vi "Main.vi"(11 "Module Admin":refnum<class "Delacor_lib_QMH_Module Admin.lvclass">) -> ()   [LabVIEW 2020, in "User Interface.lvlib"]
doc: "This template is based off of the Queued Message Handler design pattern and the Queued Message Handler project template that ships with LabVIEW.\n\nThe main difference is that the queue is private to this module and communication between modules is performed via Broadcast and Request events.\n\nRequest events are wrapped in public API methods and are handled in the Event Handling Loop (EHL) of this VI. Any module can register for Broadcast events sent by this module. The EHL generates messages based on user interface actions.\n\nThe Message Handling Loop (MHL) processes messages generated by the EHL, or by other messages. The messages are string values, so new messages can be added easily to the Message Cases case structure in the MHL. Each message cluster can also provide an optional value for Message Data, which is a variant that can be converted to whatever message-specific data is required.\n_____\nBased on DQMH Project Template 6.1.0.94."
uses:
  User Interface.lvlib
  <vilib>/Delacor/Delacor QMH/Libraries/Module Admin_class/Delacor_lib_QMH_Module Admin.lvclass
  Module Data--cluster.ctl
  Stop Argument--cluster.ctl
  <vilib>/Delacor/Delacor QMH/Libraries/Message Queue_class/Delacor_lib_QMH_Message Queue.lvclass/Delacor_lib_QMH_Message Queue.ctl
  <vilib>/Delacor/Delacor QMH/Libraries/Module Admin_class/Delacor_lib_QMH_Module Admin.lvclass/Delacor_lib_QMH_Module Admin.ctl
  <vilib>/Delacor/Delacor QMH/Libraries/Message Queue_class/Delacor_lib_QMH_Enqueue Message (Single).vi
  <vilib>/Delacor/Delacor QMH/Libraries/Module Admin_class/Delacor_lib_QMH_Get External Launch.vi
  <vilib>/Utility/error.llb/Error Cluster From Error Code.vi
  <vilib>/ErrorRing/Error Ring.xnode
  <vilib>/Delacor/Delacor QMH/Libraries/Message Queue_class/Delacor_lib_QMH_Message Queue.lvclass
  Interface Change/Interface Change.lvlib
panel:
  in  "Close Panel Interface CH":bool
  in  "Open Panel Interface CH":bool
  in  "Color Box":u32(colorbox)
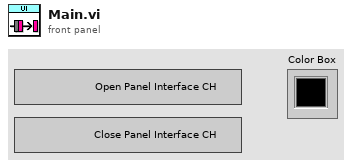
[diagram p1: front panel]
types:
  T1 = typedef "User Interface.lvlib/Request Events--cluster.ctl" = cluster{"Stop Module":refnum<user-event>, "Show Panel":refnum<user-event>, "Hide Panel":refnum<user-event>, "Get Module Execution Status":refnum<user-event>, "Show Diagram":refnum<user-event>}
  T2 = typedef "Interface Change.lvlib/Broadcast Events--cluster.ctl" = cluster{"Module Did Init":refnum<user-event>, "Status Updated":refnum<user-event>, "Error Reported":refnum<user-event>, "Module Did Stop":refnum<user-event>, "Update Module Execution Status":refnum<user-event>}
  T3 = typedef "User Interface.lvlib/Module Data--cluster.ctl" = cluster{"Status":string}
  T4 = enum32{"invalid lock state", "Not Locked", "Locked (No Password)", "Password-protected"}
  T5 = typedef "User Interface.lvlib/Stop Argument--cluster.ctl" = cluster{"Origin":string, "Exit via Stop Module Req?":bool, "Wait for Module to stop?":bool}
  T6 = enum32{"Invalid", "Standard", "Closed", "Hidden", "Minimized", "Maximized"}
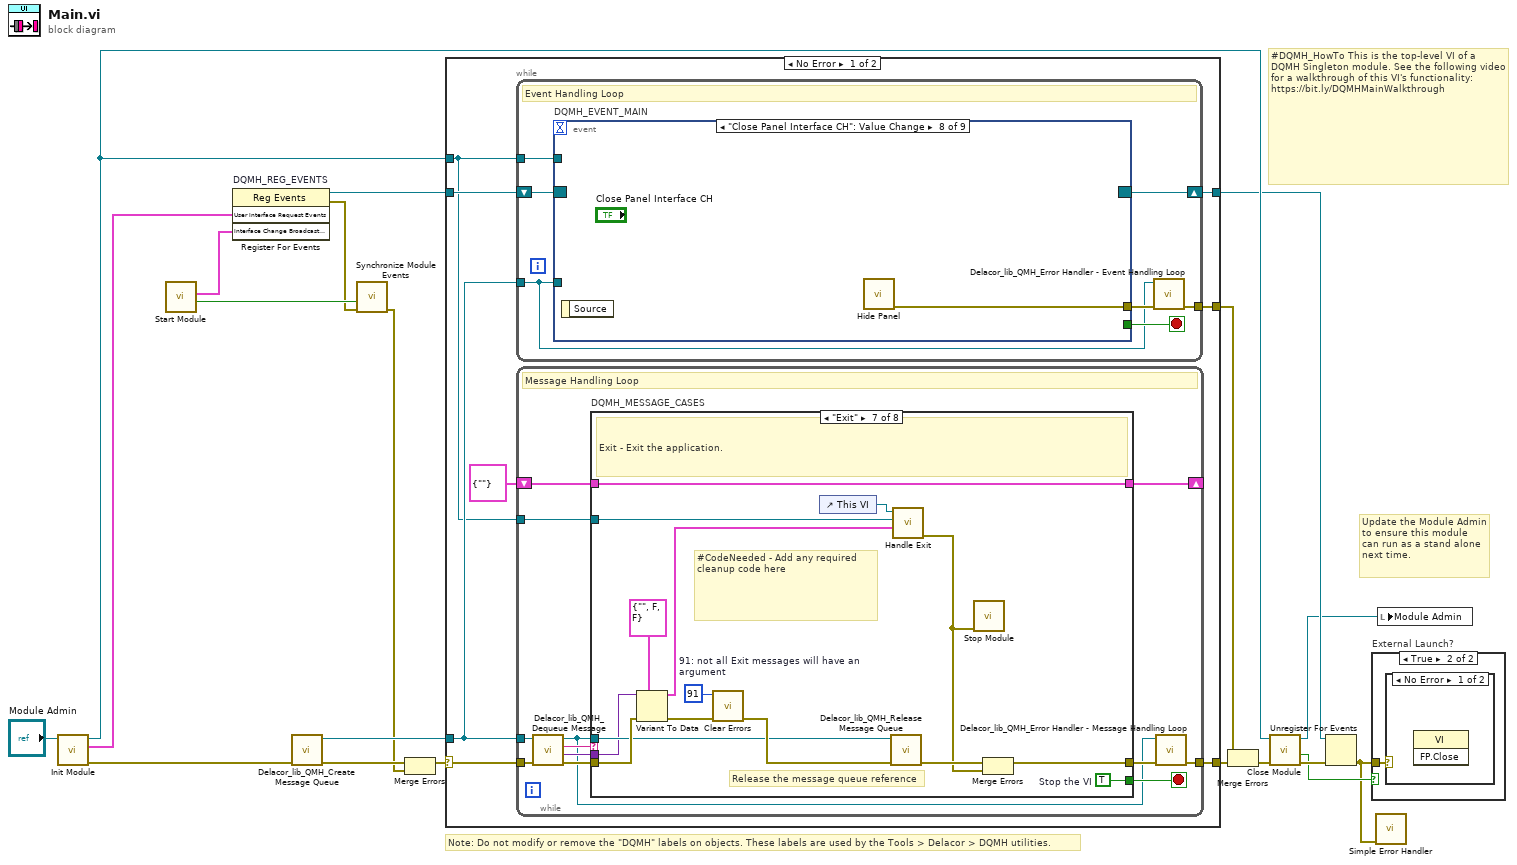
[diagram p0: block diagram]
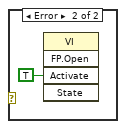
[diagram p3: hidden frame]
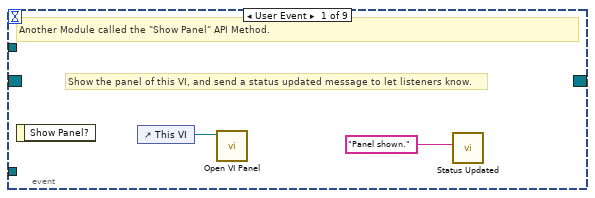
[diagram p4: hidden frame]
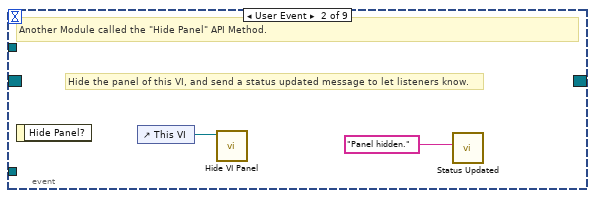
[diagram p5: hidden frame]
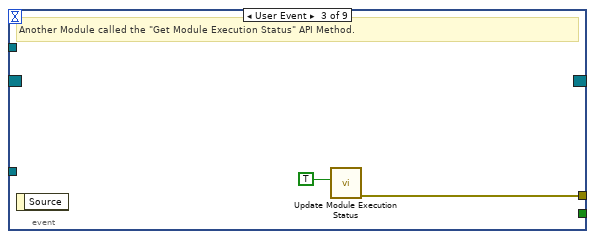
[diagram p6: hidden frame]
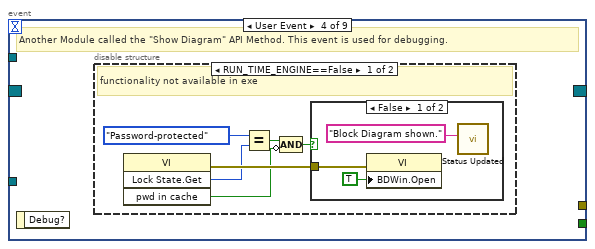
[diagram p7: hidden frame]
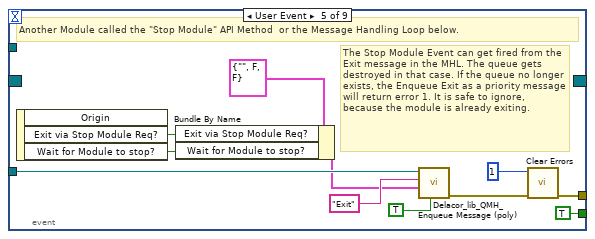
[diagram p10: hidden frame]
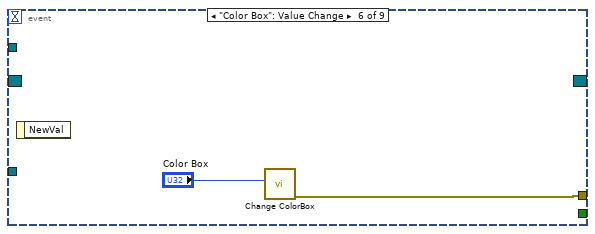
[diagram p11: hidden frame]
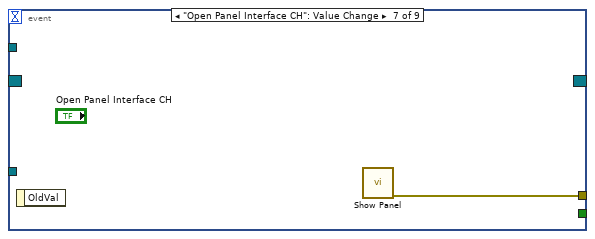
[diagram p12: hidden frame]
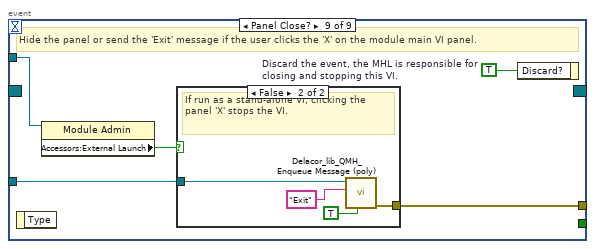
[diagram p13: hidden frame]
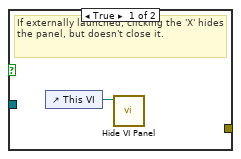
[diagram p14: hidden frame]
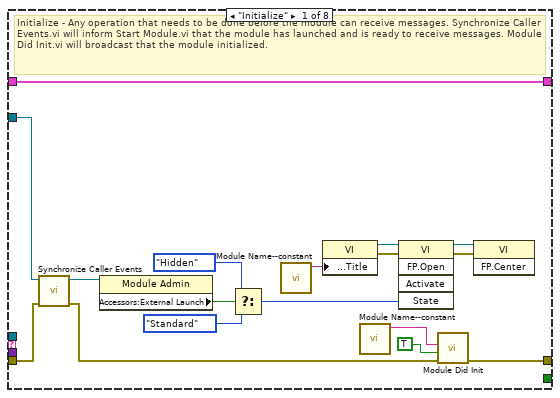
[diagram p15: hidden frame]
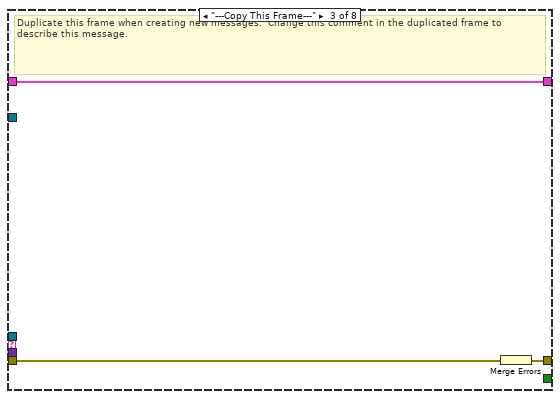
[diagram p17: hidden frame]
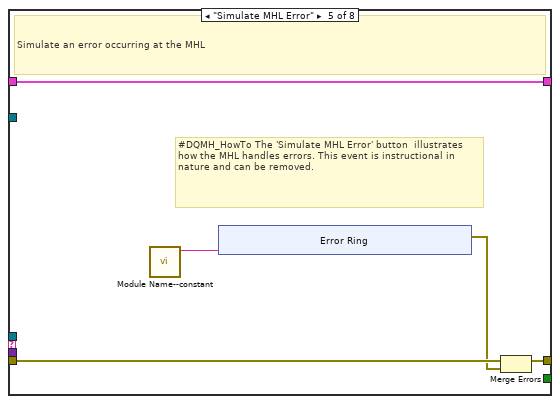
[diagram p19: hidden frame]
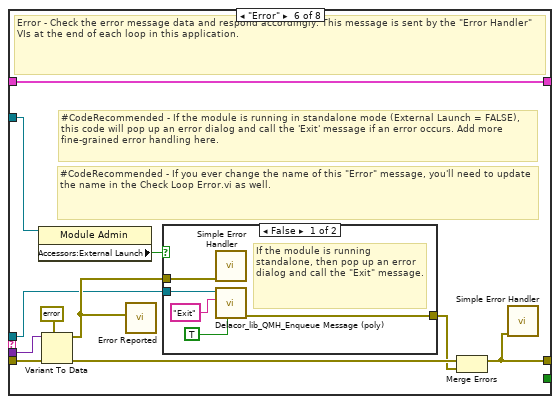
[diagram p20: hidden frame]
diagram:
  # "#DQMH_HowTo This is the top-level VI of a DQMH Singleton module. See the following video for a walkthrough of this VI's functionality: https://bit.ly/DQMHMainWalkthrough"
  # "Note: Do not modify or remove the \"DQMH\" labels on objects. These labels are used by the Tools > Delacor > DQMH utilities."
  # "Update the Module Admin to ensure this module can run as a stand alone next time."
  n1 = call "Init Module.vi"("Singleton Module Admin in"="Module Admin") -> ("error out"=w19:errorcluster, "User Interface Request Events"=w10:T1, "Singleton Module Admin out"=w13:refnum<class "Delacor_lib_QMH_Module Admin.lvclass">)  [unwired: 8 in]
  n2 = call "Start Module.vi"() -> ("Wait for Event Sync?"=w3:bool, "Interface Change Broadcast Events"=w4:T2)  [unwired: 8 in, 2 out]
  n3 = register-events "DQMH_REG_EVENTS"(w10, w4) -> (reference out=w11:refnum<event-registration>, error out=w2:errorcluster)  [unwired: 2 in]
  n4 = call <vilib>:"Delacor_lib_QMH_Create Message Queue.vi"("error in"=w19) -> ("error out"=w15:errorcluster, "Message Queue"=w9:refnum<class "Delacor_lib_QMH_Message Queue.lvclass">)  [unwired: 9 in]
  n5 = call "Synchronize Module Events.vi"("error in"=w2, "Wait for Event Sync?"=w3) -> ("error out"=w1:errorcluster)  [unwired: 9 in]
  n6 = Merge Errors(w15, w1) -> (w14:errorcluster)
  n7 = case shown="No Error" w14 {
    selector: w14 -> [w26 w171]
    tunnel: [w28 w170] -> w20
    tunnel: [w25 w176] -> w12
    tunnel: w11 -> [w23 w176]
    tunnel: w9 -> [w22 w169]
    tunnel: [w27 _] -> w17
    tunnel: w13 -> [w21 w172]
    frame No Error {
      n8 = while {
        tunnel: w22 -> [w29]
        shift-right: [w32] -> w25
        shift-left: w23 -> [w33]
        tunnel: [w34] -> w27
        tunnel: w21 -> [w30]
        stop <- w31 stop-if-true
        # "Event Handling Loop"
        n9 = event "DQMH_EVENT_MAIN" shown="[7] \"Close Panel Interface CH\": Value Change" {
          selector: w33 -> [_ _ _ _ _ _ _ _ _]
          dyn-events: [_ _ _ _ _ _ _ _ _] -> w32
          timeout: _ -> [_ _ _ _ _ _ _ _ _]
          tunnel: [_ _ _ _ TRUE ("Discard?") _ _ _ _] -> w31
          tunnel: w29 -> [_ _ _ _ w57 _ _ _ w68]
          tunnel: [_ _ w41 _ w60 w63 w64 w65 w70] -> w35
          tunnel: w30 -> [_ _ _ _ _ _ _ _ w67]
          event User Event {
            # "Show the panel of this VI, and send a status updated message to let listeners know."
            # "Another Module called the \"Show Panel\" API Method."
            n10 = event-data() -> ()  [unwired: 1 in, 1 out]
            n11 = control-ref of="This VI"() -> (w37:refnum<vi>)
            n12 = call "Open VI Panel.vi"("VI"=w37) -> ()  [unwired: 10 in, 1 out]
            n13 = call "Status Updated.vi"("Status"="Panel shown." ("format string")) -> ()  [unwired: 10 in, 1 out]
          }
          event User Event {
            # "Hide the panel of this VI, and send a status updated message to let listeners know."
            # "Another Module called the \"Hide Panel\" API Method."
            n14 = event-data() -> ()  [unwired: 1 in, 1 out]
            n15 = control-ref of="This VI"() -> (w39:refnum<vi>)
            n16 = call "Hide VI Panel.vi"("VI"=w39) -> ()  [unwired: 10 in, 1 out]
            n17 = call "Status Updated.vi"("Status"="Panel hidden." ("format string")) -> ()  [unwired: 10 in, 1 out]
          }
          event User Event {
            # "Another Module called the \"Get Module Execution Status\" API Method."
            n18 = event-data() -> ()  [unwired: 1 in, 1 out]
            n19 = call "Update Module Execution Status.vi"("Running?"=TRUE) -> ("error out"=w41:errorcluster)  [unwired: 10 in]
          }
          event User Event {
            # "Another Module called the \"Show Diagram\" API Method. This event is used for debugging."
            n20 = event-data() -> ()  [unwired: 1 in, 1 out]
            n21 = disable-structure shown="RUN_TIME_ENGINE==False" {
              frame condition #0 (active) {
                # "functionality not available in exe"
                n22 = invoke class="VI" method="Lock State.Get"() -> (error out=w47:errorcluster, "Get Lock State"=w46:T4, "pwd in cache"=w43:bool)  [unwired: 4 in, 1 out]
                n23 = Equal?(x=T4."Password-protected", y=w46) -> (x = y?=w44:bool)
                n24 = Compound Arithmetic op=AND(w44, invert w43) -> (w42:bool)
                n25 = case shown="False" w42 {
                  tunnel: w47 -> [w50 _]
                  frame False {
                    n26 = property class="VI"(error in=w50, "BDWin.Open"=TRUE ("Block Diagram Window:Open")) -> ()  [unwired: 1 in, 2 out]
                    n27 = call "Status Updated.vi"("Status"="Block Diagram shown." ("format string")) -> ()  [unwired: 10 in, 1 out]
                  }
                  frame True {
                    # "Password-protected VI, and the password is not in the cache. Do not show the diagram."
                  }
                }
              }
              frame condition #1 {
              }
            }
          }
          event User Event {
            # "The Stop Module Event can get fired from the Exit message in the MHL. The queue gets destroyed in that case. If the queue no longer exists, the Enqueue Exit as a priority message will return error 1. It is safe to ignore, because the module is already exiting."
            # "Another Module called the \"Stop Module\" API Method  or the Message Handling Loop below."
            n28 = event-data() -> ("Exit via Stop Module Req?"=w53:bool, "Wait for Module to stop?"=w52:bool)  [unwired: 1 in, 1 out]
            n29 = Bundle By Name(cluster=T5 {"Origin"="", "Exit via Stop Module Req?"=FALSE, "Wait for Module to stop?"=FALSE} ("Stop Argument"), "Exit via Stop Module Req?"=w53, "Wait for Module to stop?"=w52) -> (w51:T5)
            n30 = call-poly <vilib>:"Delacor_lib_QMH_Enqueue Message (poly).vi"("Priority Message? (F)"=TRUE, "Message Data"=w51, "Message"="Exit", "Message Queue in"=w57) -> ("error out"=w61:errorcluster)  [unwired: 6 in, 1 out]
            n31 = call <vilib>:"Clear Errors.vi"("error in (no error)"=w61, "specific error code to clear (0: all)"=1) -> ("error out"=w60:errorcluster)  [unwired: 4 in, 1 out]
          }
          event "Color Box": Value Change {
            n32 = event-data() -> ()  [unwired: 1 in, 1 out]
            n33 = call "Change ColorBox.vi"("Color Box"="Color Box") -> ("error out"=w63:errorcluster)  [unwired: 10 in]
          }
          event "Open Panel Interface CH": Value Change {
            n34 = event-data() -> ()  [unwired: 1 in, 1 out]
            n35 = call "Show Panel.vi"() -> ("error out"=w64:errorcluster)  [unwired: 11 in]
          }
          event "Close Panel Interface CH": Value Change {
            n36 = event-data() -> ()  [unwired: 1 in, 1 out]
            n37 = call "Hide Panel.vi"() -> ("error out"=w65:errorcluster)  [unwired: 11 in]
          }
          event Panel Close? {
            w69 = TRUE  # Discard the event, the MHL is responsible for closing and stopping this VI.
            # "Hide the panel or send the 'Exit' message if the user clicks the 'X' on the module main VI panel."
            n38 = event-data() -> ()  [unwired: 1 in, 1 out]
            n39 = property class="Module Admin"(reference=w67) -> ("Accessors:External Launch"=w66:bool)  [unwired: 1 in, 2 out]
            n40 = case shown="False" w66 {
              tunnel: w68 -> [_ w74]
              tunnel: [_ w75] -> w70
              frame True {
                # "If externally launched, clicking the 'X' hides the panel, but doesn't close it."
                n41 = control-ref of="This VI"() -> (w71:refnum<vi>)
                n42 = call "Hide VI Panel.vi"("VI"=w71) -> ()  [unwired: 10 in, 1 out]
              }
              frame False {
                # "If run as a stand-alone VI, clicking the panel 'X' stops the VI."
                n43 = call-poly <vilib>:"Delacor_lib_QMH_Enqueue Message (poly).vi"("Priority Message? (F)"=TRUE, "Message"="Exit", "Message Queue in"=w74) -> ("error out"=w75:errorcluster)  [unwired: 7 in, 1 out]
              }
            }
            n44 = event-data("Discard?"=w69) -> ()  [unwired: 1 in, 1 out]
          }
        }
        n45 = call-dynamic "Delacor_lib_QMH_Error Handler - Event Handling Loop.vi"("error in"=w35, "Message Queue in"=w29) -> ("dup error in"=w34:errorcluster)  [unwired: 8 in, 1 out]
      }
      n46 = while {
        tunnel: w22 -> [w78]
        shift-right: [w82] -> _
        shift-left: T3 {"Status"=""} ("Data Cluster") -> [w83]
        tunnel: w26 -> [w86]
        tunnel: [w84] -> w28
        tunnel: w21 -> [w76]
        stop <- w81 stop-if-true
        # "Message Handling Loop"
        n47 = call-dynamic "Delacor_lib_QMH_Dequeue Message.vi"("error in"=w86, "Message Queue in"=w78) -> ("error out"=w85:errorcluster, "Message Data"=w79:variant, "Message"=w80:string, "Message Queue out"=w77:refnum<class "Delacor_lib_QMH_Message Queue.lvclass">)  [unwired: 6 in]
        n48 = case "DQMH_MESSAGE_CASES" shown="\"Exit\"" w80 {
          selector: w80 -> [_ _ _ _ _ _ _ w156]
          tunnel: w77 -> [_ _ _ _ _ w127 w149 _]
          tunnel: w85 -> [w102 w106 w109 w111 w116 w133 w154 w158]
          tunnel: [w100 w106 w108 w111 w115 w124 w151 w159] -> w87
          tunnel: w83 -> [w88 w105 w107 w110 w113 w129 w148 w157]
          tunnel: [w88 w105 w107 w110 w113 w129 w148 w157] -> w82
          tunnel: [_ _ _ _ _ _ w147 _] -> w81
          tunnel: w79 -> [_ _ _ _ _ w128 w146 _]
          tunnel: w76 -> [w92 _ _ _ _ w126 w141 _]
          frame "Initialize" {
            # "Initialize - Any operation that needs to be done before the module can receive messages. Synchronize Caller Events.vi will inform Start Module.vi that the module has launched and is ready to receive messages. Module Did Init.vi will broadcast that the module initialized."
            n49 = call "Synchronize Caller Events.vi"("error in (no error)"=w102, "Singleton Module Admin in"=w92) -> ("error out"=w101:errorcluster, "Singleton Module Admin out"=w89:refnum<class "Delacor_lib_QMH_Module Admin.lvclass">)  [unwired: 8 in]
            n50 = property class="Module Admin"(reference=w89) -> ("Accessors:External Launch"=w96:bool)  [unwired: 1 in, 2 out]
            n51 = Select(t=T6."Hidden" ("State"), s=w96, f=T6."Standard" ("State")) -> (s? t:f=w93:T6)
            n52 = call "Module Name--constant.vi"() -> ("Module Name"=w99:string)  [unwired: 11 in]
            n53 = property class="VI"("Front Panel.Title"=w99) -> (reference out=w98:refnum<vi>, error out=w104:errorcluster)  [unwired: 2 in]
            n54 = call "Module Name--constant.vi"() -> ("Module Name"=w90:string)  [unwired: 11 in]
            n55 = invoke class="VI" method="FP.Open"(reference=w98, error in=w104, "State"=w93) -> (reference out=w97:refnum<vi>, error out=w103:errorcluster)  [unwired: 2 in, 3 out]
            n56 = call "Module Did Init.vi"("error in (no error)"=w101, "Initialized?"=TRUE, "Origin"=w90) -> ("error out"=w100:errorcluster)  [unwired: 8 in]
            n57 = invoke class="VI" method="FP.Center"(reference=w97, error in=w103) -> ()  [unwired: 1 in, 3 out]
          }
          frame "---Module Specific---" {
            # "Separator -- The following cases handle messages specific to this Module."
          }
          frame "---Copy This Frame---" {
            # "Duplicate this frame when creating new messages.  Change this comment in the duplicated frame to describe this message."
            n58 = Merge Errors(w109) -> (w108:errorcluster)
          }
          frame "---Exit and Error Handling---" {
            # "Separator - The following cases handle errors and exit messages."
          }
          frame "Simulate MHL Error" {
            # "#DQMH_HowTo The 'Simulate MHL Error' button  illustrates how the MHL handles errors. This event is instructional in nature and can be removed."
            # "Simulate an error occurring at the MHL"
            n59 = call "Module Name--constant.vi"() -> ("Module Name"=w112:string)  [unwired: 11 in]
            n60 = xnode "Error Ring"("parameter 0"=w112) -> ("error out"=w114:errorcluster)
            n61 = Merge Errors(w116, w114) -> (w115:errorcluster)
          }
          frame "Error" {
            # "#CodeRecommended - If you ever change the name of this \"Error\" message, you'll need to update the name in the Check Loop Error.vi as well."
            # "#CodeRecommended - If the module is running in standalone mode (External Launch = FALSE), this code will pop up an error dialog and call the 'Exit' message if an error occurs. Add more fine-grained error handling here."
            # "Error - Check the error message data and respond accordingly. This message is sent by the \"Error Handler\" VIs at the end of each loop in this application."
            n62 = property class="Module Admin"(reference=w126) -> ("Accessors:External Launch"=w125:bool)  [unwired: 1 in, 2 out]
            n63 = Variant To Data(error in=w133, type=errorcluster {"status"=FALSE, "code"=0, "source"=""} ("error constant"), Variant=w128) -> (data=w134:errorcluster, error out=w131:errorcluster)
            n64 = call "Error Reported.vi"("Error"=w134) -> ()  [unwired: 10 in, 1 out]
            n65 = case shown="False" w125 {
              tunnel: [w139 _] -> w130
              tunnel: w127 -> [w137 _]
              tunnel: w134 -> [w138 _]
              frame False {
                # "If the module is running standalone, then pop up an error dialog and call the \"Exit\" message."
                n66 = call <vilib>:"Simple Error Handler.vi"("error in (no error)"=w138) -> ()  [unwired: 4 in, 5 out]
                n67 = call-poly <vilib>:"Delacor_lib_QMH_Enqueue Message (poly).vi"("Priority Message? (F)"=TRUE, "Message"="Exit", "Message Queue in"=w137) -> ("error out"=w139:errorcluster)  [unwired: 7 in, 1 out]
              }
              frame True {
                # "If the module was launched externally, calling the Error Reported broadcast VI is the only action performed by the \"Error\" message. The module's caller can then process the error appropriately."
              }
            }
            n68 = Merge Errors(w131, w130) -> (w124:errorcluster)
            n69 = call <vilib>:"Simple Error Handler.vi"("error in (no error)"=w124) -> ()  [unwired: 4 in, 5 out]
          }
          frame "Exit" {
            w145 = 91  # 91: not all Exit messages will have an argument
            w147 = TRUE  # Stop the VI
            # "Release the message queue reference"
            # "#CodeNeeded - Add any required cleanup code here"
            # "Exit - Exit the application."
            n70 = Variant To Data(error in=w154, type=T5 {"Origin"="", "Exit via Stop Module Req?"=FALSE, "Wait for Module to stop?"=FALSE} ("Stop Argument"), Variant=w146) -> (data=w143:T5, error out=w150:errorcluster)
            n71 = call <vilib>:"Clear Errors.vi"("error in (no error)"=w150, "specific error code to clear (0: all)"=w145) -> ("error out"=w153:errorcluster)  [unwired: 4 in, 1 out]
            n72 = control-ref of="This VI"() -> (w142:refnum<vi>)
            n73 = call-dynamic "Delacor_lib_QMH_Release Message Queue.vi"("error in"=w153, "Message Queue"=w149) -> ("error out"=w152:errorcluster)  [unwired: 9 in]
            n74 = call "Handle Exit.vi"("Stop Argument"=w143, "Admin in"=w141, "VI reference"=w142) -> ("error out"=w140:errorcluster)  [unwired: 7 in, 1 out]
            n75 = call "Stop Module.vi"("error in"=w140) -> ()  [unwired: 10 in, 1 out]
            n76 = Merge Errors(w152, w140) -> (w151:errorcluster)
          }
          frame Default {
            # "'Default' case only runs if there is a message that isn't defined in any of the other cases.  Output a programming error."
            n77 = call "Module Name--constant.vi"() -> ("Module Name"=w155:string)  [unwired: 11 in]
            n78 = xnode "Error Ring"("parameter 0"=w156, "parameter 1"=w155) -> ("error out"=w160:errorcluster)
            n79 = Merge Errors(w158, w160) -> (w159:errorcluster)
          }
        }
        n80 = call-dynamic "Delacor_lib_QMH_Error Handler - Message Handling Loop.vi"("error in"=w87, "Message Queue in"=w77) -> ("dup error in"=w84:errorcluster)  [unwired: 8 in, 1 out]
      }
    }
    frame Error {
      # "Synchronize Caller Events.vi will inform Start Module.vi that the module has launched and will let the code calling Start Module.vi register for broadcasts and would permit the caller receive the broadcast that an error occurred at launch time."
      n81 = call-dynamic "Delacor_lib_QMH_Release Message Queue.vi"("error in"=w171, "Message Queue"=w169) -> ("error out"=w170:errorcluster)  [unwired: 9 in]
      n82 = call "Synchronize Caller Events.vi"("Singleton Module Admin in"=w172) -> ("error out"=w177:errorcluster)  [unwired: 9 in, 1 out]
      n83 = call "Module Name--constant.vi"() -> ("Module Name"=w175:string)  [unwired: 11 in]
      n84 = Format Into String(format string="An error occurred during initialization. %s is no longer running.", w175) -> (resulting string=w173:string)  [unwired: 2 in, 1 out]
      n85 = Merge Errors(w170, w177) -> (w178:errorcluster)
      n86 = call "Error Reported.vi"("Additional Information"=w173, "Error"=w178) -> ()  [unwired: 9 in, 1 out]
    }
  }
  n87 = Merge Errors(w17, w20) -> (w16:errorcluster)
  n88 = call "Close Module.vi"("error in (no error)"=w16, "Module Admin in"=w13) -> ("error out"=w18:errorcluster, "External Launch"=w6:bool, "Module Admin out"=w7:refnum<class "Delacor_lib_QMH_Module Admin.lvclass">)  [unwired: 7 in]
  n89 = Unregister For Events(event registration refnum=w12, error in=w18) -> (error out=w5:errorcluster)
  n90 = case "External Launch?" shown="True" w6 {
    tunnel: w5 -> [_ w179]
    frame False {
    }
    frame True {
      n91 = case shown="No Error" w179 {
        frame No Error {
          n92 = invoke class="VI" method="FP.Close"() -> ()  [unwired: 3 in, 3 out]
        }
        frame Error {
          n93 = invoke class="VI" method="FP.Open"("Activate"=TRUE ("Activate?")) -> ()  [unwired: 4 in, 5 out]
        }
      }
    }
  }
  n94 = call <vilib>:"Simple Error Handler.vi"("error in (no error)"=w5) -> ()  [unwired: 4 in, 5 out]
  n95 = local write "Module Admin"(w7) -> ()
